vi "Write data bits.vi"(8 "error in (no error)":errorcluster, 10 "data bits":u16=8, 11 "Serial Master in":refnum<class "Serial Interface.lvclass">) -> (0 "error out":errorcluster, 3 "Serial Master out":refnum<class "Serial Interface.lvclass">)   [LabVIEW 2021, in "Serial Interface.lvclass"]
uses:
  Serial Interface.lvclass
  Serial Interface.lvclass/Serial Interface.ctl
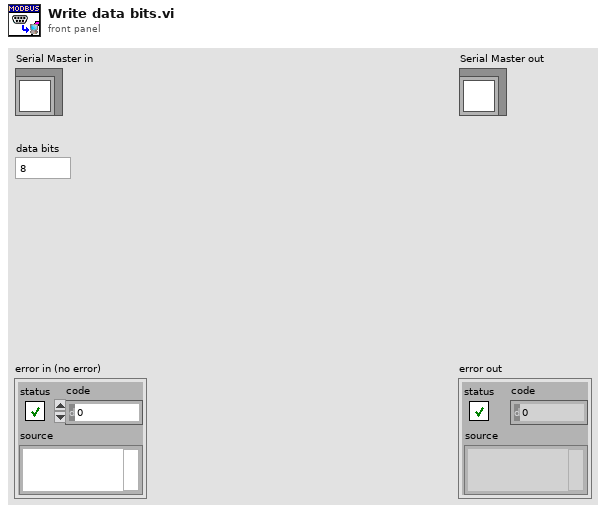
[diagram p1: front panel]
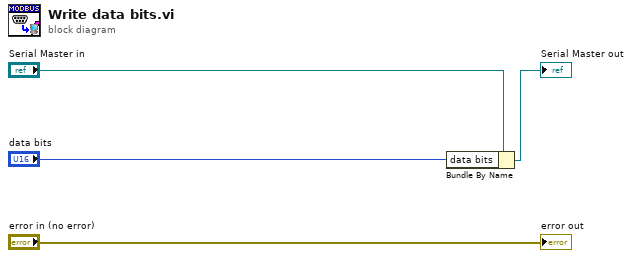
[diagram p0: block diagram]
diagram:
  n1 = Bundle By Name(cluster="Serial Master in", "data bits"="data bits") -> (→"Serial Master out":refnum<class "Serial Interface.lvclass">)
  "error out" <- "error in (no error)"
